vi "Remove Task Request.vi"(8 "error in (no error)":errorcluster, 10 "Task":variant, 11 "BuildWorker in":refnum<class "BuildWorker.lvclass">) -> (0 "error out":errorcluster, 3 "BuildWorker out":refnum<class "BuildWorker.lvclass">)   [LabVIEW 2017, in "BuildWorker.lvlib" / "BuildWorker.lvclass"]
uses:
  BuildWorker.lvclass
  Classes/Task Interface/Task/Task.lvclass
  Classes/Task Interface/Task/Status.ctl
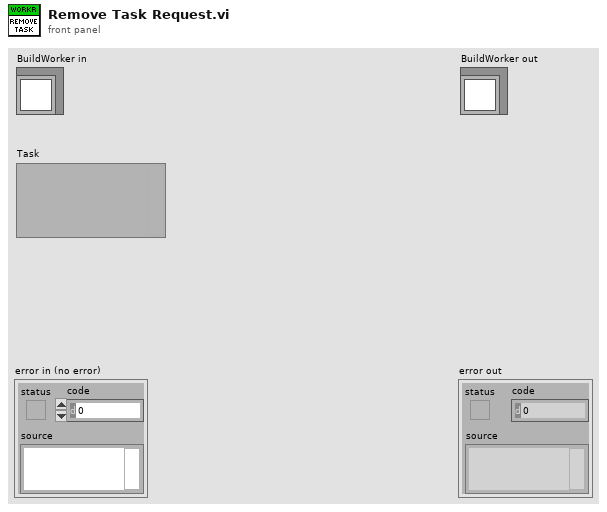
[diagram p1: front panel]
types:
  T1 = typedef "Task Interface.lvlib/Task.lvclass/Status.ctl" = enum16{"Created", "Added", "Pending", "Queued", "Processing", "Cleaning", "Building", "Finished", "Failed", "Removed", "Not found"}
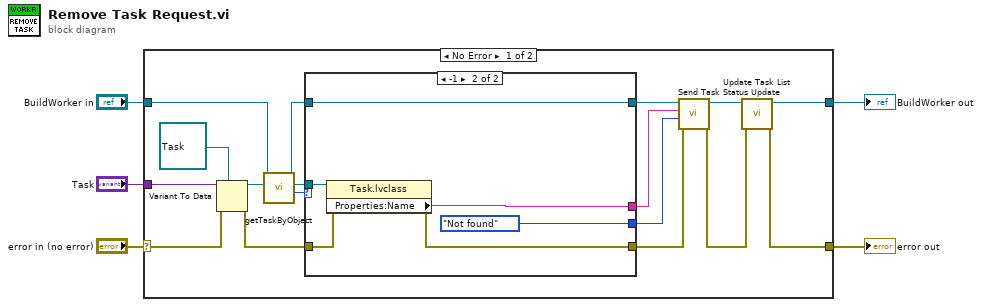
[diagram p0: block diagram]
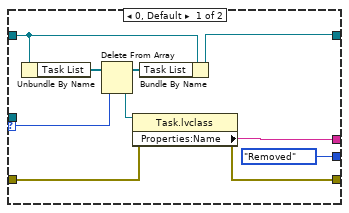
[diagram p2: hidden frame]
diagram:
  n1 = case shown="No Error" "error in (no error)" {
    selector: "error in (no error)" -> [w21 w40]
    tunnel: [w18 w40] -> w4
    tunnel: [w19 w39] -> w2
    tunnel: "BuildWorker in" -> [w17 w39]
    tunnel: "Task" -> [w22 _]
    frame No Error {
      n2 = Variant To Data(error in=w21, type=refnum<class "Task.lvclass"> refnum ("Task Interface.lvlib:Task.lvclass"), Variant=w22) -> (data=w16:refnum<class "Task.lvclass">, error out=w20:errorcluster)
      n3 = call "getTaskByObject.vi"("Task Object"=w16, "BuildWorker in"=w17) -> ("index of element"=w15:i32, "Task"=w7:refnum<class "Task.lvclass">, "BuildWorker out"=w14:refnum<class "BuildWorker.lvclass">)  [unwired: 7 in]
      n4 = case shown="-1" w15 {
        selector: w15 -> [w32 _]
        tunnel: [w30 w35] -> w9
        tunnel: w20 -> [w31 w36]
        tunnel: [w29 w38] -> w11
        tunnel: w14 -> [w27 w37]
        tunnel: [w26 w37] -> w13
        tunnel: [Status."Removed" ("Status") Status."Not found" ("Status")] -> w10
        tunnel: w7 -> [_ w33]
        frame 0, Default {
          n5 = Unbundle By Name(w27) -> ("Task List"=w28:refnum<class "Task.lvclass">[])
          n6 = Delete From Array(array=w28, index=w32) -> (deleted portion=w24:refnum<class "Task.lvclass">, array with subset deleted=w25:refnum<class "Task.lvclass">[])  [unwired: 1 in]
          n7 = property class="Task.lvclass"(reference=w24, error in=w31) -> (error out=w30:errorcluster, "Properties:Name"=w29:string)  [unwired: 1 out]
          n8 = Bundle By Name(cluster=w27, "Task List"=w25) -> (w26:refnum<class "BuildWorker.lvclass">)
        }
        frame -1 {
          n9 = property class="Task.lvclass"(reference=w33, error in=w36) -> (error out=w35:errorcluster, "Properties:Name"=w38:string)  [unwired: 1 out]
        }
      }
      n10 = call "Send Task Status Update.vi"("error in (no error)"=w9, "Status"=w10, "Task Name"=w11, "BuildWorker in"=w13) -> ("error out"=w8:errorcluster, "BuildWorker out"=w12:refnum<class "BuildWorker.lvclass">)  [unwired: 6 in]
      n11 = call "Update Task List.vi"("error in (no error)"=w8, "BuildWorker in"=w12) -> ("error out"=w18:errorcluster, "BuildWorker out"=w19:refnum<class "BuildWorker.lvclass">)  [unwired: 8 in]
    }
    frame Error {
    }
  }
  "error out" <- w4
  "BuildWorker out" <- w2
